vi "util_PhotodiodeCalibration-ViP.vi"(10 "Laser":enum16{"473nm", "532nm"}(ring), 11 "Ai":i32) -> (3 "P (mW)":dbl)   [LabVIEW 2012]
uses:
  <vilib>/Analysis/NI_AALPro.lvlib
panel:
  out "Power (mW) vs. Voltage":cluster{dbl[], dbl[]}[](graph)
  out "intercept":dbl
  out "slope":dbl
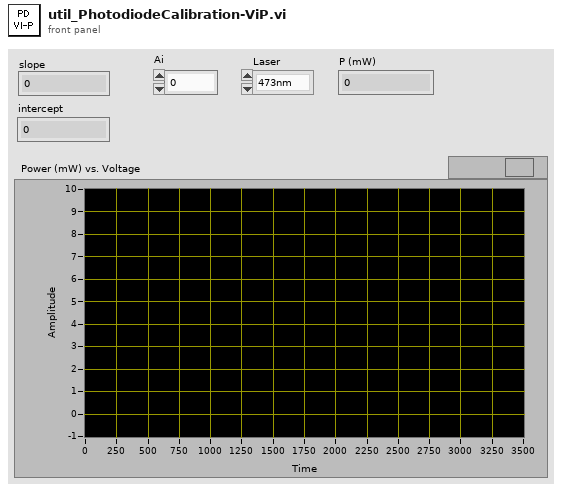
[diagram p1: front panel]
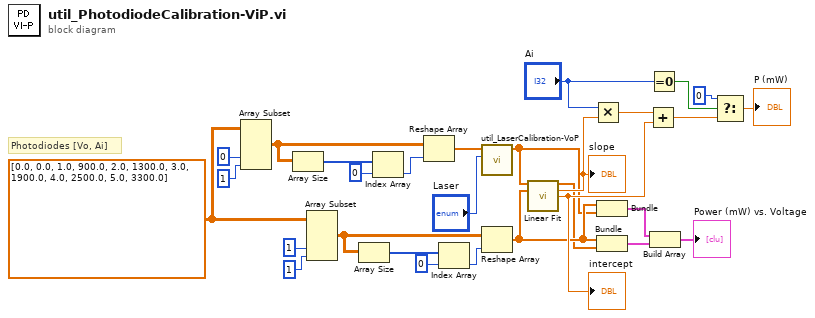
[diagram p0: block diagram]
diagram:
  w17 = dbl[][] [[0.0, 0.0], [1.0, 900.0], [2.0, 1300.0], [3.0, 1900.0], [4.0, 2500.0], [5.0, 3300.0]]
  # "Photodiodes [Vo, Ai]"
  n1 = Array Subset(array=w17, index (col)=0 ("index"), length (col)=1 ("length")) -> (w24:dbl[][])  [unwired: 2 in]
  n2 = Array Size(array=w24) -> (size(s)=w26:i32[])
  n3 = Array Subset(array=w17, index (col)=1 ("index"), length (col)=1 ("length")) -> (w18:dbl[][])  [unwired: 2 in]
  n4 = Array Size(array=w18) -> (size(s)=w20:i32[])
  n5 = Index Array(array=w26, index=0) -> (element=w25:i32)
  n6 = Reshape Array(w24, w25) -> (w14:dbl[])
  n7 = Index Array(array=w20, index=0) -> (element=w19:i32)
  n8 = call "util_LaserCalibration-VoP.vi"("Vo"=w14, "Laser"="Laser") -> ("P (mW)"=w1:dbl[])  [unwired: 8 in]
  n9 = Reshape Array(w18, w19) -> (w10:dbl[])
  n10 = call <vilib>:"Linear Fit.vi"("Y"=w1, "X"=w10) -> ("Best Linear Fit"=w9:dbl[], "slope"=w16:dbl, "intercept"=w15:dbl)  [unwired: 9 in, 2 out]
  "slope" <- w16
  "intercept" <- w15
  n11 = Multiply(x="Ai", y=w16) -> (x*y=w13:dbl)
  n12 = Bundle(w10, "P (mW)"=w1) -> (w7:cluster{dbl[], "P (mW)":dbl[]})  [unwired: 1 in]
  n13 = Bundle(w10, "Best Linear Fit"=w9) -> (w8:cluster{dbl[], "Best Linear Fit":dbl[]})  [unwired: 1 in]
  n14 = Add(x=w13, y=w15) -> (x+y=w3:dbl)
  n15 = Equal To 0?(x="Ai") -> (x = 0?=w5:bool)
  n16 = Build Array(w7, w8) -> (→"Power (mW) vs. Voltage":cluster{dbl[], "Best Linear Fit":dbl[]}[])
  n17 = Select(t=0 ("length"), s=w5, f=w3) -> (s? t:f=→"P (mW)":dbl)
